vi "crop_image_dimension_to_SLM_size.vi"(9 "max size":dbl, 11 "original size":dbl) -> (1 "end index":u16, 3 "start index":u16)   [LabVIEW 2025]
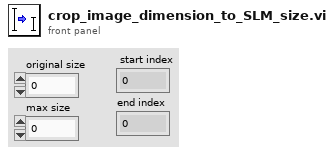
[diagram p1: front panel]
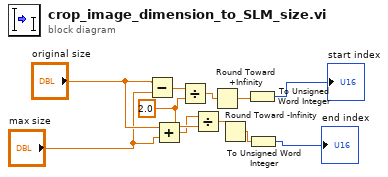
[diagram p0: block diagram]
diagram:
  w8 = 2.0 ("y")
  n1 = Subtract(x="original size", y="max size") -> (x-y=w11:dbl)
  n2 = Add(x="original size", y="max size") -> (x+y=w7:dbl)
  n3 = Divide(x=w11, y=w8) -> (x/y=w10:dbl)
  n4 = Divide(x=w7, y=w8) -> (x/y=w6:dbl)
  n5 = Round Toward +Infinity(x=w10) -> (ceil(x): smallest int >= x=w9:dbl)
  n6 = Round Toward -Infinity(1:w6) -> (0:w5:dbl)
  n7 = To Unsigned Word Integer(number=w9) -> (unsigned 16bit integer=→"start index":u16)
  n8 = To Unsigned Word Integer(number=w5) -> (unsigned 16bit integer=→"end index":u16)
